vi "Module Name--constant.vi"() -> (3 "Module Name":string)   [LabVIEW 2015, in "Thermal Chamber Controller_DQMH.lvlib"]
doc: "Return the name of the module that owns this VI. \n_____\nBased on Delacor QMH Project Template 2.0.0.62.\n____\nDelacor QMH Thermal Chamber Examples 4.0.0.21\nCopyright (c) 2018, Delacor"
uses:
  Thermal Chamber Controller_DQMH.lvlib
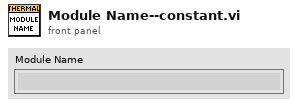
[diagram p1: front panel]
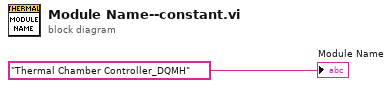
[diagram p0: block diagram]
diagram:
  "Module Name" <- "Thermal Chamber Controller_DQMH"
